vi "Configure Q-Switch State.vi"(7 "Q-switch (primary)":u16(ring)=1 items=["primary"=1, "secondary"=2], 8 "error in (no error)":errorcluster, 10 "on":bool, 11 "Lotis in":refnum<class "PL Lotis TII LS.lvclass">) -> (0 "error out":errorcluster, 3 "Lotis out":refnum<class "PL Lotis TII LS.lvclass">)   [LabVIEW 2015, in "PL Lotis TII LS.lvclass"]
doc: "Configures Q-switch state."
uses:
  PL Lotis TII LS.lvclass
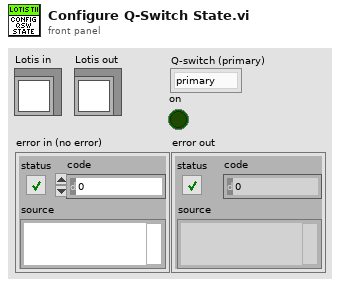
[diagram p1: front panel]
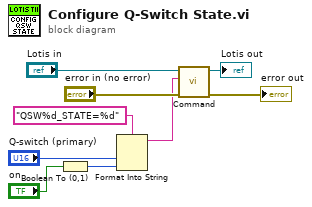
[diagram p0: block diagram]
diagram:
  n1 = Boolean To (0,1)(Boolean="on") -> (0, 1=w1:i16)
  n2 = Format Into String(format string="QSW%d_STATE=%d" ("command"), "Q-switch (primary)", w1) -> (resulting string=w4:string)  [unwired: 2 in, 1 out]
  n3 = call "Command.vi"("error in (no error)"="error in (no error)", "command"=w4, "Lotis in"="Lotis in") -> ("error out"=→"error out":errorcluster, "Lotis out"=→"Lotis out":refnum<class "PL Lotis TII LS.lvclass">)  [unwired: 6 in, 1 out]
